vi "Read Stim Mode Labels (SubVI).vi"(11 "STIM MODE":string) -> (3 "Label":string[](array[string]))   [LabVIEW 2020]
uses:
  <vilib>/Utility/file.llb/Read Delimited Spreadsheet (string).vi
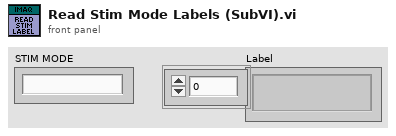
[diagram p1: front panel]
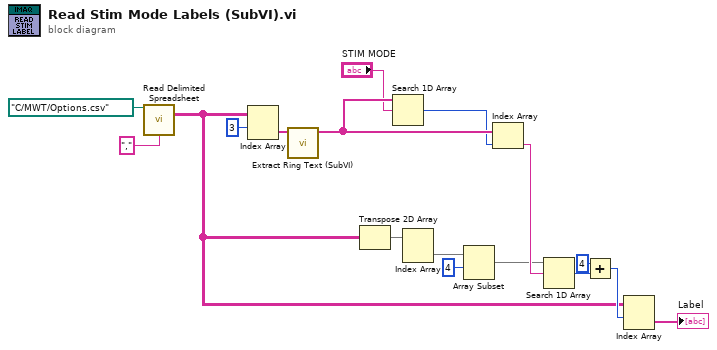
[diagram p0: block diagram]
diagram:
  n1 = call-poly <vilib>:"Read Delimited Spreadsheet.vi"("file path (dialog if empty)"=path "C:/MWT/Options.csv", "delimiter (\\t)"="," ("delimiter (\\t)")) -> ("all rows"=w13:string[][])  [unwired: 8 in, 5 out]
  n2 = Index Array(array=w13, index (row)=3) -> (element=w4:string[])  [unwired: 1 in]
  n3 = call "Extract Ring Text (SubVI).vi"("Spreadsheet String"=w4) -> ("Output String"=w3:string[])  [unwired: 10 in]
  n4 = Transpose 2D Array(2D array=w13) -> (transposed array=w8:string[][])
  n5 = Search 1D Array(1D array=w3, element="STIM MODE") -> (index of element=w1:i32)  [unwired: 1 in]
  n6 = Index Array(array=w8) -> (element=w9:string[])  [unwired: 2 in]
  n7 = Array Subset(array=w9, index=4) -> (w11:string[])  [unwired: 1 in]
  n8 = Index Array(array=w3, index=w1) -> (element=w12:string)
  n9 = Search 1D Array(1D array=w11, element=w12) -> (index of element=w14:i32)  [unwired: 1 in]
  n10 = Add(x=4, y=w14) -> (x+y=w15:i32)
  n11 = Index Array(array=w13, index (row)=w15) -> (element=→"Label":string[])  [unwired: 1 in]
